vi "ep_Complete Voltage Event.vi"(0 "time":timestamp, 1 "event type":T3, 5 "voltage RMS":dbl, 7 "phase":T2, 9 "event state":T1(ring), 11 "dt":dbl=0.01) -> (4 "voltage events":T4(array[cluster]))   [LabVIEW 2011, in "NI_EP_Power Quality.lvlib"]
uses:
  <vilib>/addons/Electrical Power/PQ/NI_EP_Power Quality.lvlib
  <vilib>/addons/Electrical Power/PQ/Common/Controls/ep_Event Type.ctl
  <vilib>/addons/Electrical Power/PQ/Common/Controls/ep_Phase.ctl
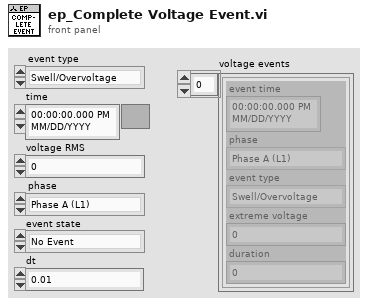
[diagram p1: front panel]
types:
  T1 = enum16{"No Event", "Begin of Event", "End of Event", "Event in progress"}
  T2 = typedef "NI_EP_Power Quality.lvlib/ep_Phase.ctl" = enum16{"Phase A (L1)", "Phase B (L2)", "Phase C (L3)", "Phase N", "~3 Phases"}
  T3 = typedef "NI_EP_Power Quality.lvlib/ep_Event Type.ctl" = enum16{"Swell/Overvoltage", "Dip/Undervoltage", "Interruption"}
  T4 = cluster{"event time":timestamp, "phase":T2, "event type":T3, "extreme voltage":dbl, "duration":dbl}[]
  T5 = cluster{"event time":timestamp, "phase":T2, "event type":T3, "extreme voltage":dbl, "duration":dbl}
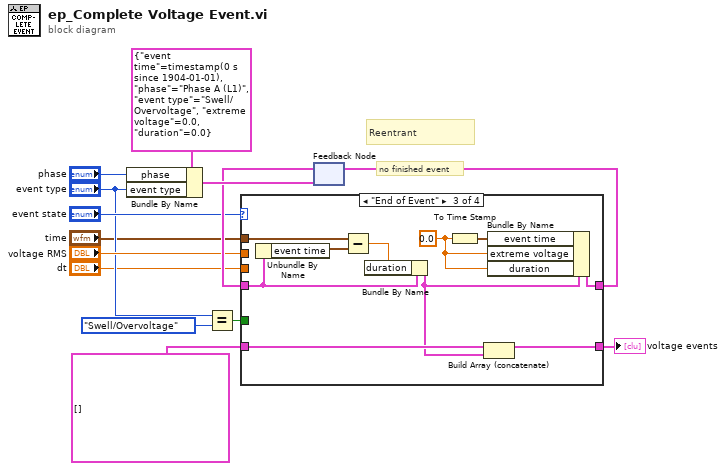
[diagram p0: block diagram]
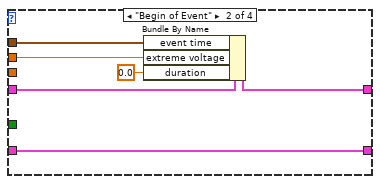
[diagram p3: hidden frame]
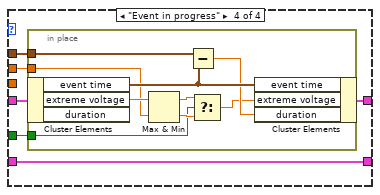
[diagram p4: hidden frame]
diagram:
  # "Reentrant"
  # "no finished event"
  n1 = Bundle By Name(cluster=T5 {"event time"=timestamp(0 s since 1904-01-01), "phase"=enum."Phase A (L1)", "event type"=enum."Swell/Overvoltage", "extreme voltage"=0.0, "duration"=0.0} ("voltage event"), "phase"="phase", "event type"="event type") -> (w12:T5)
  n2 = Equal?(x="event type", y=ep_Event_Type."Swell/Overvoltage") -> (x = y?=w8:bool)
  n3 = feedback #1(w12) -> (w11:T5)
  n4 = case shown="\"End of Event\"" "event state" {
    tunnel: "time" -> [_ w17 w27 w38]
    tunnel: "voltage RMS" -> [_ w22 _ w37]
    tunnel: w8 -> [_ _ _ w36]
    tunnel: T4 [] ("voltage events") -> [w16 w21 w32 w35]
    tunnel: [w16 w21 w31 w35] -> w14
    tunnel: [w15 w20 w30 w34] -> w3
    tunnel: w11 -> [w15 w19 w25 w33]
    tunnel: "dt" -> [_ _ _ _]
    frame "No Event", Default {
    }
    frame "Begin of Event" {
      n5 = Bundle By Name(cluster=w19, "event time"=w17, "extreme voltage"=w22, "duration"=0.0) -> (w20:T5)
    }
    frame "End of Event" {
      w28 = 0.0
      n6 = Unbundle By Name(w25) -> ("event time"=w26:timestamp)
      n7 = Subtract(x=w27, y=w26) -> (x-y=w24:dbl)
      n8 = Bundle By Name(cluster=w25, "duration"=w24) -> (w23:T5)
      n9 = To Time Stamp(1:w28) -> (0:w29:timestamp)
      n10 = Build Array (concatenate)(w32, w23) -> (w31:T4)
      n11 = Bundle By Name(cluster=w23, "event time"=w29, "extreme voltage"=w28, "duration"=w28) -> (w30:T5)
    }
    frame "Event in progress" {
      n12 = in-place {
        in-place-border: w38 -> [w47]
        in-place-border: w37 -> [w43]
        in-place-border: w36 -> [w39]
        n13 = in-place-cluster #2(w33) -> ("event time"=w46:timestamp, "extreme voltage"=w44:dbl)  [unwired: 1 out]
        n14 = Max & Min(x=w44, y=w43) -> (max(x,y)=w42:dbl, min(x,y)=w41:dbl)
        n15 = Subtract(x=w47, y=w46) -> (x-y=w45:dbl)
        n16 = Select(t=w42, s=w39, f=w41) -> (s? t:f=w40:dbl)
        n17 = in-place-cluster #2("event time"=w46, "extreme voltage"=w40, "duration"=w45) -> (w34:T5)
      }
    }
  }
  "voltage events" <- w14
  n18 = feedback-in #1(w3) -> ()
